vi "rs3 get device count2.vi"(8 "error in":errorcluster, 11 "device_list":u64) -> (0 "error out":errorcluster, 1 "device_list_out":u64, 2 "device count":i32, 3 "error":u64)   [LabVIEW 2018, in "libRealSense3.lvlib"]
doc: "Determine number of connected DEVICES. \nEach device will have many sensors. \n \nINPUT: \ndevice list Input handle from QUERY DEVICES call.\n\nOUTPUT: \nDevice count Number of device attached\nError 0=no error"
uses:
  libRealSense3.lvlib
  realsense2.dll
panel:
  # "RS3 Get Device Count2"
  # "(C) Intel Corp.,  AGJ"
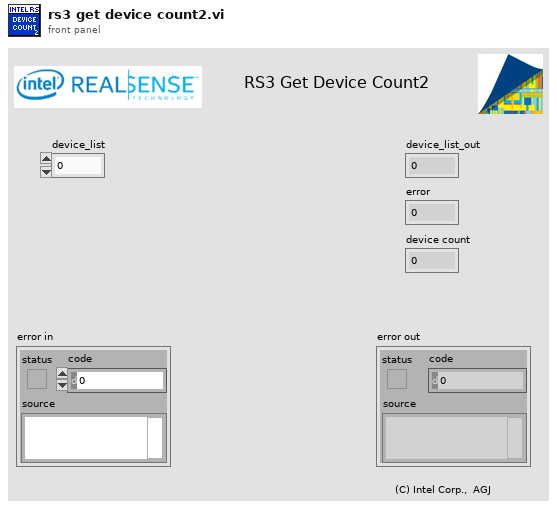
[diagram p1: front panel]
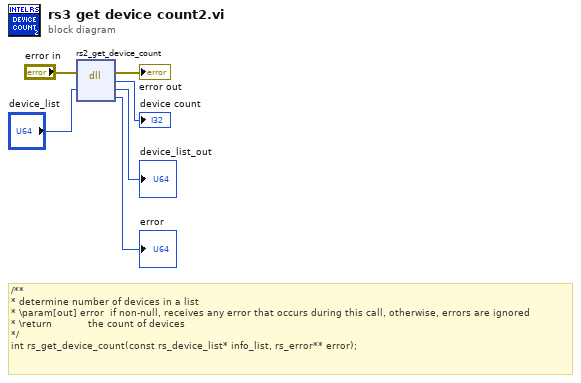
[diagram p0: block diagram]
diagram:
  # "/**\n* determine number of devices in a list\n* \\param[out] error  if non-null, receives any error that occurs during this call, otherwise, errors are ignored\n* \\return            the count of devices\n*/\nint rs_get_device_count(const rs_device_list* info_list, rs_error** error);"
  n1 = dll-call lib="C:/Users/aaron.jencks/Documents/Temp/realsense_labview_sdk/RealSense SDK2.11.0 for LabVIEW/realsense2.dll" fn="rs2_get_device_count"(error in="error in", "device list"="device_list") -> (error out=→"error out":errorcluster, "device count"=→"device count":i32, "device list"=→"device_list_out":u64, "error"=→"error":u64)  [unwired: 3 in, 1 out]
